vi "P4CMDSub Convert Opened List to Array.vi"(4 "opened string":string) -> (1 "changelist files array":string[](array[string]))   [LabVIEW 2020, in "NI_SCC_P4CMD.lvlib"]
uses:
  <vilib>/SourceControl/Providers/P4CMD/NI_SCC_P4CMD.lvlib
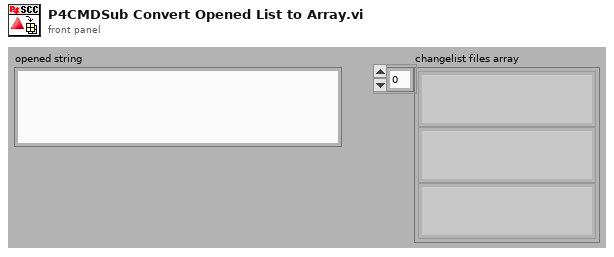
[diagram p1: front panel]
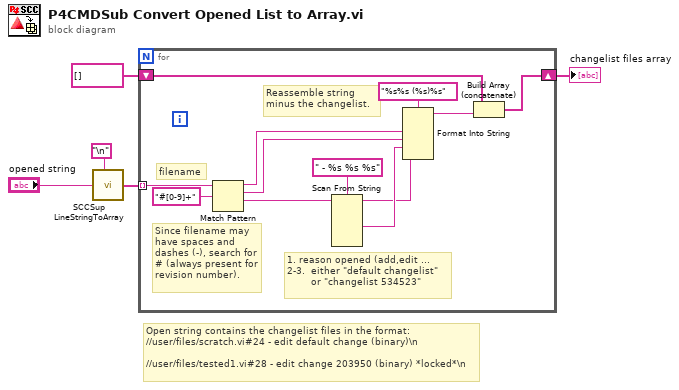
[diagram p0: block diagram]
diagram:
  # "Open string contains the changelist files in the format:\n//user/files/scratch.vi#24 - edit default change (binary)\\n\n\n//user/files/tested1.vi#28 - edit change 203950 (binary) *locked*\\n"
  n1 = call <vilib>:"SCCSup LineStringToArray.vi"("delimiter (Tab)"="\n", "line string"="opened string") -> ("line array"=w3:string[])  [unwired: 7 in]
  n2 = for {
    tunnel: w3 -> [w8] mode=indexing
    shift-right: [w6] -> w1
    shift-left: string[] [] -> [w7]
    # "1. reason opened (add,edit ...\n2-3.  either \"default changelist\"\n        or \"changelist 534523\""
    # "Reassemble string\nminus the changelist."
    # "Since filename may have spaces and dashes (-), search for # (always present for revision number)."
    # "filename"
    n3 = Match Pattern(string=w8, regular expression="#[0-9]+") -> (before substring=w13:string, match substring=w12:string, after substring=w15:string)  [unwired: 1 in, 1 out]
    n4 = Scan From String(format string=" - %s %s %s", input string=w15) -> (remaining string=w10:string, output 1=w11:string)  [unwired: 7 in, 2 out]
    n5 = Format Into String(format string="%s%s (%s)%s", w13, w12, w11, w10) -> (resulting string=w9:string)  [unwired: 2 in, 1 out]
    n6 = Build Array (concatenate)(w7, w9) -> (w6:string[])
  }
  "changelist files array" <- w1
